vi "Create.vi"(8 "error in":errorcluster, 11 "34972A in":refnum<class "34972A.lvclass">) -> (0 "error out":errorcluster, 3 "34972A out":refnum<class "34972A.lvclass">)   [LabVIEW 2020, in "34972A.lvclass"]
uses:
  34972A.lvclass
  34972A.lvclass/34972A.ctl
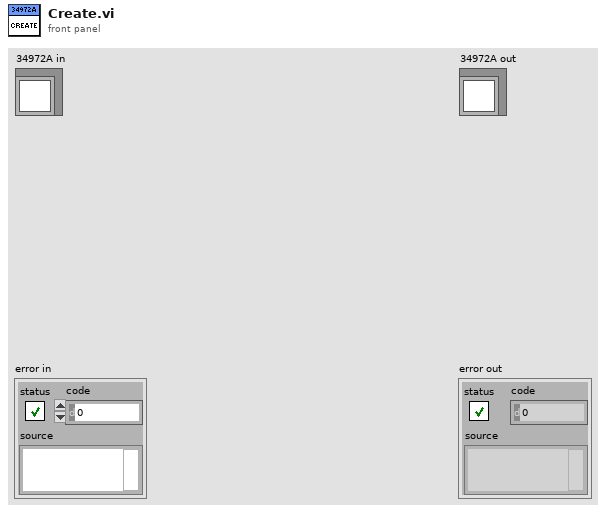
[diagram p1: front panel]
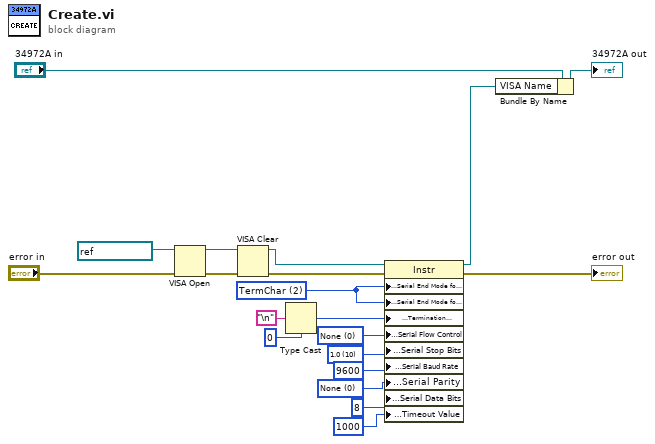
[diagram p0: block diagram]
diagram:
  w10 = u16 0 items=["None", "XON/XOFF", "RTS/CTS", "XON/XOFF & RTS/CTS", "DTR/DSR", "XON/XOFF & DTR/DSR"] ("Serial Settings:Flow Control")
  w13 = u16 0 items=["None", "Odd", "Even", "Mark", "Space"] ("Serial Settings:Serial Parity")
  w14 = u16 10 items=["1.0"=10, "1.5"=15, "2.0"=20] ("Serial Settings:Serial Stop Bits")
  w18 = u16 2 items=["None", "LastBit", "TermChar"] ("Serial Settings:Serial End Mode for Reads")
  n1 = VISA Open(error in (no error)="error in", VISA resource name=refnum<visa-resource-name> "Firstborn") -> (VISA resource name=w20:refnum<visa-resource-name>, error out=w19:errorcluster)  [unwired: 3 in]
  n2 = VISA Clear(VISA resource name=w20, error in (no error)=w19) -> (VISA resource name out=w1:refnum<visa-resource-name>, error out=w5:errorcluster)
  n3 = Type Cast(type=u8 0, x="\n" ("Line Feed Constant")) -> (*(type *) &x=w15:u8)
  n4 = property on="Property Node" class="Instr"(reference=w1, error in=w5, "Serial Settings:Serial End Mode for Reads"=w18, "Serial Settings:Serial End Mode for Writes"=w18, "Message Based Settings:Termination Character"=w15, "Serial Settings:Serial Flow Control"=w10, "Serial Settings:Serial Stop Bits"=w14, "Serial Settings:Serial Baud Rate"=u32 9600 ("Serial Settings:Baud Rate"), "Serial Settings:Serial Parity"=w13, "Serial Settings:Serial Data Bits"=u16 8, "General Settings:Timeout Value"=u32 1000) -> (reference out=w2:refnum<visa-resource-name>, error out=→"error out":errorcluster)
  n5 = Bundle By Name(cluster="34972A in", "VISA Name"=w2) -> (→"34972A out":refnum<class "34972A.lvclass">)
